vi "Read Troque.vi"(0 "reference in":refnum<class "SmartMotor.lvclass">, 5 "error in (no error)":errorcluster) -> (14 "reference out":refnum<class "SmartMotor.lvclass">, 18 "Motor Torque":i32, 19 "error out":errorcluster)   [LabVIEW 2017, in "SmartMotor.lvclass"]
uses:
  SmartMotor.lvclass
  utils/SmartMotor Error.ctl
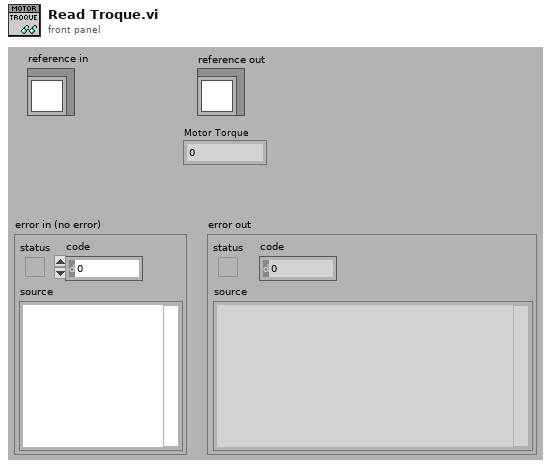
[diagram p1: front panel]
types:
  T1 = typedef "SmartMotor.lvclass/SmartMotor Error.ctl" = enum8{"None", "Read Error", "Low Voltage"}
  T2 = typedef "SmartMotor.lvclass/ObjectAttributes.ctl" = cluster{"SmartMotor Chain VISA Resource":refnum<visa-resource-name>, "SmartMotor Chain Address":i16, "Motor Absolute Position":i32, "Motor Relative Position":i32, "Motor Torque":i32, "Motor Voltage":i32, "Screwdriver Engaged":bool, "Screwdriver Torque Limit":i32, "Torque Monitor On/Off Status":bool, "Torque Monitor VI Reference":refnum<vi>, "Absolute Motor Torque (Filtered)":dbl, "SmartMotor Status":T3, "SmartMotor Error":T1}
  T3 = typedef "SmartMotor.lvclass/SmartMotor Status.ctl" = enum8{"Stopped", "Moving"}
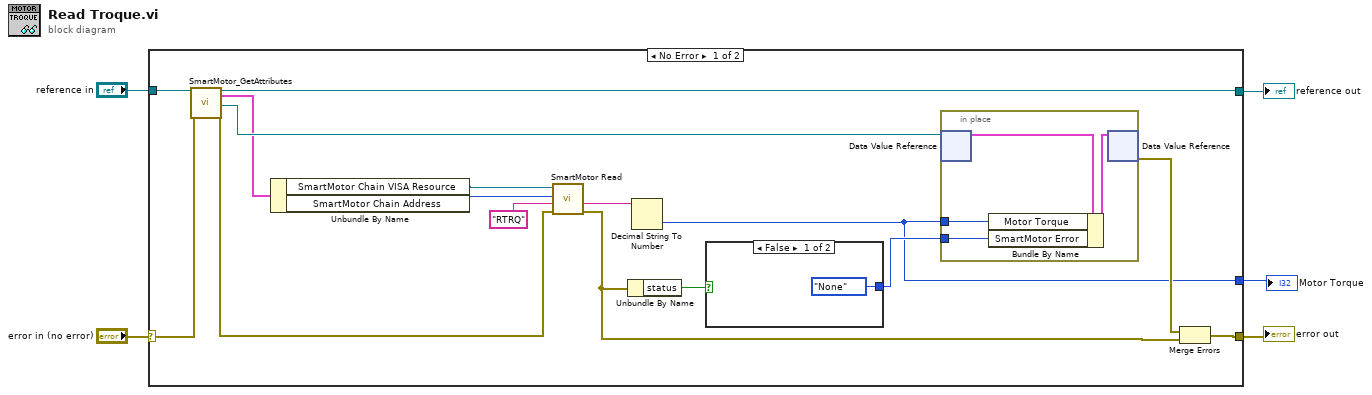
[diagram p0: block diagram]
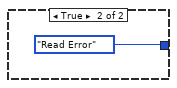
[diagram p2: hidden frame]
diagram:
  n1 = case shown="No Error" "error in (no error)" {
    selector: "error in (no error)" -> [w20 w29]
    tunnel: [w18 w29] -> w4
    tunnel: [w19 w28] -> w2
    tunnel: "reference in" -> [w21 w28]
    tunnel: [w7 _] -> w1
    frame No Error {
      n2 = call "SmartMotor_GetAttributes.vi"("reference in"=w21, "error in (no error)"=w20) -> ("reference out"=w19:refnum<class "SmartMotor.lvclass">, "Data"=w15:T2, "DataRef"=w17:refnum<data-value>, "error out"=w9:errorcluster)  [unwired: 14 in]
      n3 = Unbundle By Name(w15) -> ("SmartMotor Chain VISA Resource"=w11:refnum<visa-resource-name>, "SmartMotor Chain Address"=w10:i16)
      n4 = call "SmartMotor Read.vi"("VISA resource IN"=w11, "Motor Number"=w10, "Read Command to Motor"="RTRQ", "Error In"=w9) -> ("Response From Motor"=w13:string, "Error Out"=w6:errorcluster)  [unwired: 1 in, 3 out]
      n5 = Unbundle By Name(w6) -> ("status"=w12:bool)
      n6 = Decimal String To Number(string=w13) -> (number=w7:i32)  [unwired: 2 in, 1 out]
      n7 = case shown="False" w12 {
        tunnel: [SmartMotor_Error."None" ("SmartMotor Status") SmartMotor_Error."Read Error" ("SmartMotor Status")] -> w8
        frame False {
        }
        frame True {
        }
      }
      n8 = in-place {
        in-place-border: w7 -> [w25]
        in-place-border: w8 -> [w24]
        n9 = in-place-dvr #1(w17) -> (w26:T2)  [unwired: 1 out]
        n10 = Bundle By Name(cluster=w26, "Motor Torque"=w25, "SmartMotor Error"=w24) -> (w27:T2)
        n11 = in-place-dvr #1(w27) -> (w16:errorcluster)  [unwired: 1 out]
      }
      n12 = Merge Errors(w16, w6) -> (w18:errorcluster)
    }
    frame Error {
    }
  }
  "error out" <- w4
  "reference out" <- w2
  "Motor Torque" <- w1
